vi "RemoveFunction (SubVI).vi"(11 "Table in":refnum<vi>) -> ()   [LabVIEW 2017]
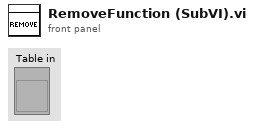
[diagram p1: front panel]
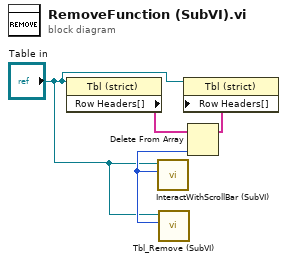
[diagram p0: block diagram]
diagram:
  n1 = property on="Property Node" class="Tbl (strict)"(reference="Table in") -> ("Row Headers[]"=w2:string[])  [unwired: 1 in, 2 out]
  n2 = call "Tbl_Remove (SubVI).vi"("Table in"="Table in") -> ("element"=w4:i32)  [unwired: 10 in]
  n3 = call "InteractWithScrollBar (SubVI).vi"("element"=w4, "Table in"="Table in") -> ()  [unwired: 10 in]
  n4 = Delete From Array(array=w2, index=w4) -> (array with subset deleted=w3:string[])  [unwired: 1 in, 1 out]
  n5 = property on="Property Node" class="Tbl (strict)"(reference="Table in", "Row Headers[]"=w3) -> ()  [unwired: 1 in, 2 out]
